vi "MapColor_ramp2Array.vi"(1 "Color 2":u32(colorbox)=16711680, 2 "Color 1":u32(colorbox), 3 "numColors":u16=85) -> (0 "appended array":u32[](array[numeric]))   [LabVIEW 2010]
panel:
  out "size(s)":i32
  out "ColorRamp":u32[](array[colorbox])
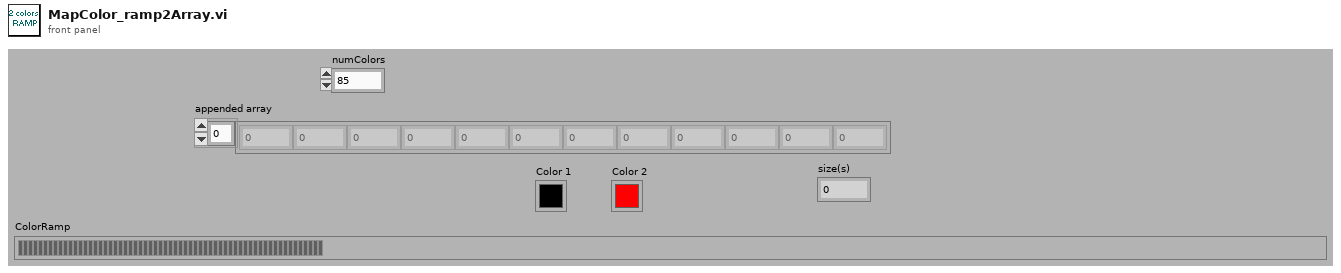
[diagram p1: front panel]
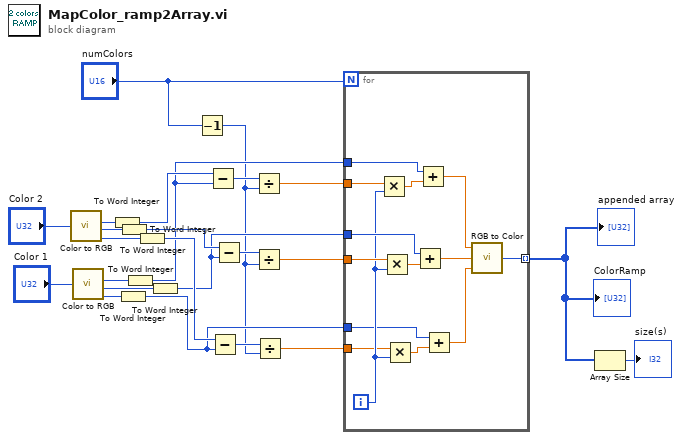
[diagram p0: block diagram]
diagram:
  n1 = call <vilib>:"Color to RGB.vi"("Color"="Color 2") -> ("R"=w11:u8, "G"=w10:u8, "B"=w9:u8)  [unwired: 1 out]
  n2 = call <vilib>:"Color to RGB.vi"("Color"="Color 1") -> ("R"=w18:u8, "G"=w16:u8, "B"=w14:u8)  [unwired: 1 out]
  n3 = To Word Integer(number=w11) -> (16bit integer=w8:i16)
  n4 = To Word Integer(number=w14) -> (16bit integer=w3:i16)
  n5 = To Word Integer(number=w10) -> (16bit integer=w7:i16)
  n6 = To Word Integer(number=w18) -> (16bit integer=w5:i16)
  n7 = To Word Integer(number=w9) -> (16bit integer=w6:i16)
  n8 = To Word Integer(number=w16) -> (16bit integer=w4:i16)
  n9 = Decrement(x="numColors") -> (x-1=w1:u16)
  n10 = Subtract(x=w8, y=w5) -> (x-y=w22:i16)
  n11 = Subtract(x=w6, y=w3) -> (x-y=w20:i16)
  n12 = Subtract(x=w7, y=w4) -> (x-y=w21:i16)
  n13 = Divide(x=w22, y=w1) -> (x/y=w19:dbl)
  n14 = Divide(x=w21, y=w1) -> (x/y=w17:dbl)
  n15 = Divide(x=w20, y=w1) -> (x/y=w15:dbl)
  n16 = for {
    N: "numColors" -> [_]
    tunnel: w19 -> [w37]
    tunnel: w5 -> [w36]
    tunnel: w17 -> [w35]
    tunnel: w4 -> [w33]
    tunnel: w15 -> [w31]
    tunnel: w3 -> [w29]
    tunnel: [w28] -> w12 mode=indexing
    i -> [w32]
    n17 = Multiply(x=w37, y=w32) -> (x*y=w38:dbl)
    n18 = Multiply(x=w35, y=w32) -> (x*y=w34:dbl)
    n19 = Multiply(x=w31, y=w32) -> (x*y=w30:dbl)
    n20 = Add(x=w33, y=w34) -> (x+y=w27:dbl)
    n21 = Add(x=w36, y=w38) -> (x+y=w25:dbl)
    n22 = Add(x=w29, y=w30) -> (x+y=w26:dbl)
    n23 = call <vilib>:"RGB to Color.vi"("B"=w26, "G"=w27, "R"=w25) -> ("Color"=w28:u32)
  }
  "appended array" <- w12
  "ColorRamp" <- w12
  n24 = Array Size(array=w12) -> (size(s)=→"size(s)":i32)
